vi "Notify Observers.vi"(8 "error in (no error)":errorcluster, 10 "Text":string, 11 "Observable in":refnum<class "Observable.lvclass">) -> (0 "error out":errorcluster, 3 "Observable out":refnum<class "Observable.lvclass">)   [LabVIEW 2011, in "Observable.lvclass"]
uses:
  Observable.lvclass
  Observable.lvclass/Observable.ctl
  Observer/Observer.lvclass
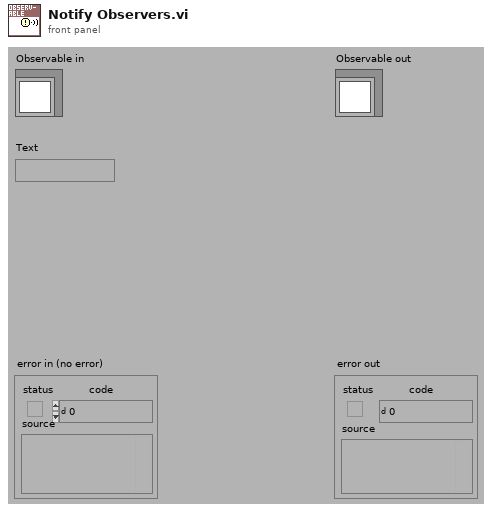
[diagram p1: front panel]
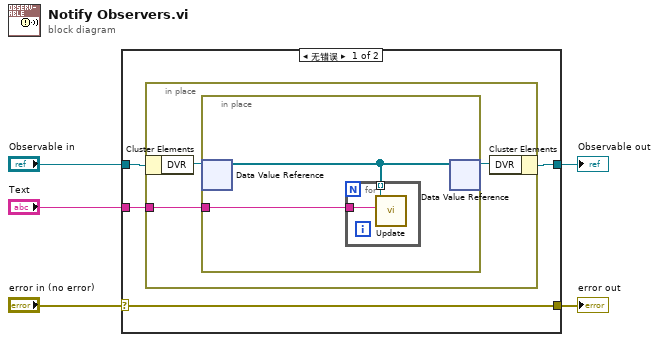
[diagram p0: block diagram]
diagram:
  n1 = case shown="无错误" "error in (no error)" {
    selector: "error in (no error)" -> [w6 w18]
    tunnel: "Observable in" -> [w9 w17]
    tunnel: [w8 w17] -> w4
    tunnel: "Text" -> [w7 _]
    tunnel: [w6 w18] -> w1
    frame No Error {
      n2 = in-place {
        in-place-border: w7 -> [w10]
        n3 = in-place-cluster #1(w9) -> ("DVR"=w12:refnum<data-value>)
        n4 = in-place {
          in-place-border: w10 -> [w13]
          n5 = in-place-dvr #2(w12) -> (w14:refnum<class "Observer.lvclass">[])  [unwired: 1 out]
          n6 = for {
            tunnel: w14 -> [w16] mode=indexing
            tunnel: w13 -> [w15]
            n7 = call-dynamic "Update.vi"("Text"=w15, "Observer in"=w16) -> ()  [unwired: 8 in, 2 out]
          }
          n8 = in-place-dvr #2(w14) -> (w11:refnum<data-value>)  [unwired: 1 out]
        }
        n9 = in-place-cluster #1("DVR"=w11) -> (w8:refnum<class "Observable.lvclass">)
      }
    }
    frame Error {
    }
  }
  "Observable out" <- w4
  "error out" <- w1
